vi "Timer_Run.vi"(8 "Stop Timer":bool, 11 "reference in":refnum<class "Timer.lvclass">) -> (3 "reference out":refnum<class "Timer.lvclass">)   [LabVIEW 2017, in "Timer.lvclass"]
uses:
  Timer.lvclass
panel:
  out "error out":errorcluster
  in  "error in (no error)":errorcluster
  # "This VI is called Asynchronously and will have one instance in memory\nfor each asynchronous call."
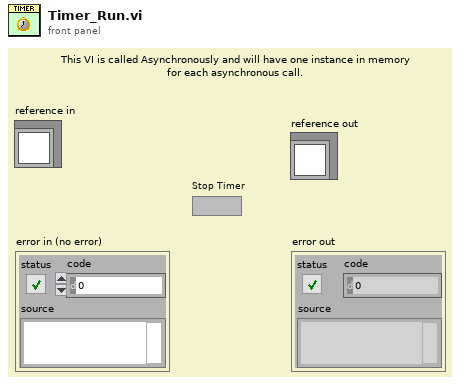
[diagram p1: front panel]
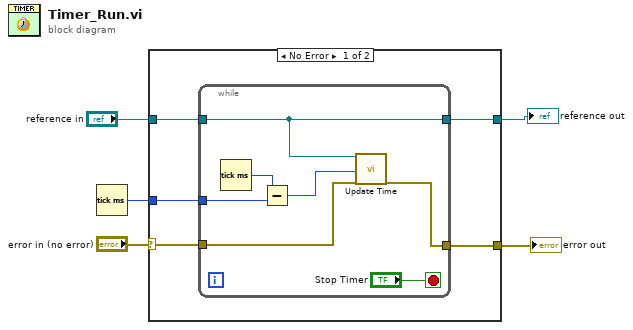
[diagram p0: block diagram]
diagram:
  n1 = Tick Count (ms)() -> (millisecond timer value=w5:u32)
  n2 = case shown="No Error" "error in (no error)" {
    selector: "error in (no error)" -> [w6 w18]
    tunnel: w5 -> [w10 _]
    tunnel: "reference in" -> [w9 _]
    tunnel: [w8 _] -> w3
    tunnel: [w7 w18] -> w2
    frame No Error {
      n3 = while {
        tunnel: w10 -> [w16]
        tunnel: w9 -> [w13]
        tunnel: [w13] -> w8
        tunnel: w6 -> [w12]
        tunnel: [w11] -> w7
        stop <- "Stop Timer" stop-if-true
        n4 = Tick Count (ms)() -> (millisecond timer value=w17:u32)
        n5 = Subtract(x=w17, y=w16) -> (x-y=w15:u32)
        n6 = call-dynamic "Update Time.vi"("reference in"=w13, "Timer Time (ms)"=w15, "error in (no error)"=w12) -> ("error out"=w11:errorcluster)  [unwired: 15 in, 1 out]
      }
    }
    frame Error {
    }
  }
  "reference out" <- w3
  "error out" <- w2
